vi "Read extParams.vi"(8 "error in":errorcluster, 11 "PAS Cell in":refnum<class "PAS Cell.lvclass">) -> (0 "error out":errorcluster, 2 "extParams":cluster{"slope":sgl, "zero":sgl}={"slope"=1.0, "zero"=0.0}, 3 "PAS Cell out":refnum<class "PAS Cell.lvclass">)   [LabVIEW 2017, in "PAS Library.lvlib" / "PAS Cell.lvclass"]
doc: "Retrieve the parameters for calculating the extinction from the integrated area.\n\next = m*IA + b"
uses:
  PAS Cell.lvclass
  PAS Cell.lvclass/PAS Cell.ctl
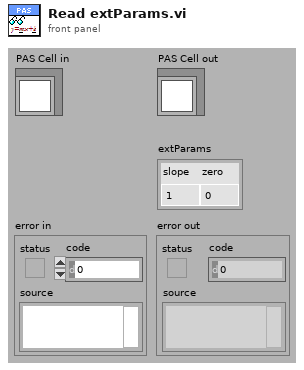
[diagram p1: front panel]
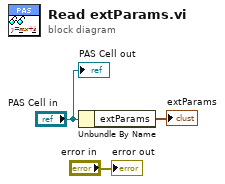
[diagram p0: block diagram]
diagram:
  n1 = Unbundle By Name("PAS Cell in") -> ("extParams"=→"extParams":cluster{"slope":sgl, "zero":sgl})
  "error out" <- "error in"
  "PAS Cell out" <- "PAS Cell in"
